vi "get channels.vi"(11 "OPC UA configuration in":refnum<class "OPC UA configuration.lvclass">) -> (2 "channels":refnum<class "TBM channel.lvclass">[](array[class]), 3 "OPC UA configuration out":refnum<class "OPC UA configuration.lvclass">)   [LabVIEW 2013, in "OPC UA configuration.lvclass"]
uses:
  OPC UA configuration.lvclass
  <vilib>/NI/Tag Bus Module Framework/channel/TBM channel.lvclass
  OPC UA configuration.lvclass/OPC UA configuration.ctl
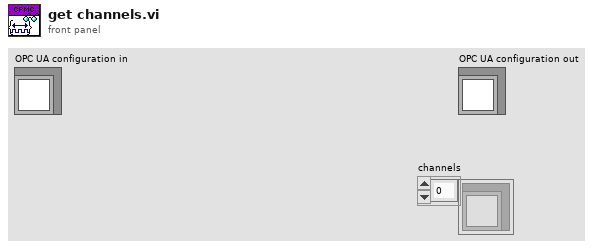
[diagram p1: front panel]
types:
  T1 = typedef "OPC UA configuration.lvclass/OPC UA Data Type.ctl" = enum16{"Bool", "SByte", "Byte", "Int16", "UInt16", "Int32", "UInt32", "Int64", "UInt64", "Float", "Double", "String", "DateTime", "ByteString", "Bool Array", "SByte Array", "Byte Array", "Int16 Array", "UInt16 Array", "Int32 Array", "UInt32 Array", "Int64 Array", "UInt64 Array", "Float Array", "Double Array", "String Array", "DateTime Array", "ByteString Array"}
  T2 = cluster{"channel":refnum<class "TBM channel.lvclass">, "Node Path":string, "OPC UA Data Type":T1}[]
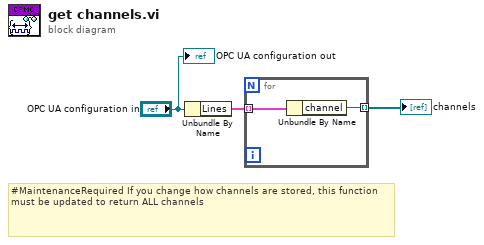
[diagram p0: block diagram]
diagram:
  # "#MaintenanceRequired If you change how channels are stored, this function must be updated to return ALL channels"
  n1 = Unbundle By Name("OPC UA configuration in") -> ("Lines"=w2:T2)
  n2 = for {
    tunnel: w2 -> [w5] mode=indexing
    tunnel: [w4] -> w1 mode=indexing
    n3 = Unbundle By Name(w5) -> ("channel"=w4:refnum<class "TBM channel.lvclass">)
  }
  "channels" <- w1
  "OPC UA configuration out" <- "OPC UA configuration in"
